vi "append_data.vi"(8 "error in (no error)":errorcluster, 10 "Current measurement #":i32, 11 "Counter in":refnum<class "Counter.lvclass">) -> (0 "error out":errorcluster, 3 "Counter out":refnum<class "Counter.lvclass">)   [LabVIEW 2013, in "Counter.lvclass"]
uses:
  Counter.lvclass
  Counter.lvclass/Counter.ctl
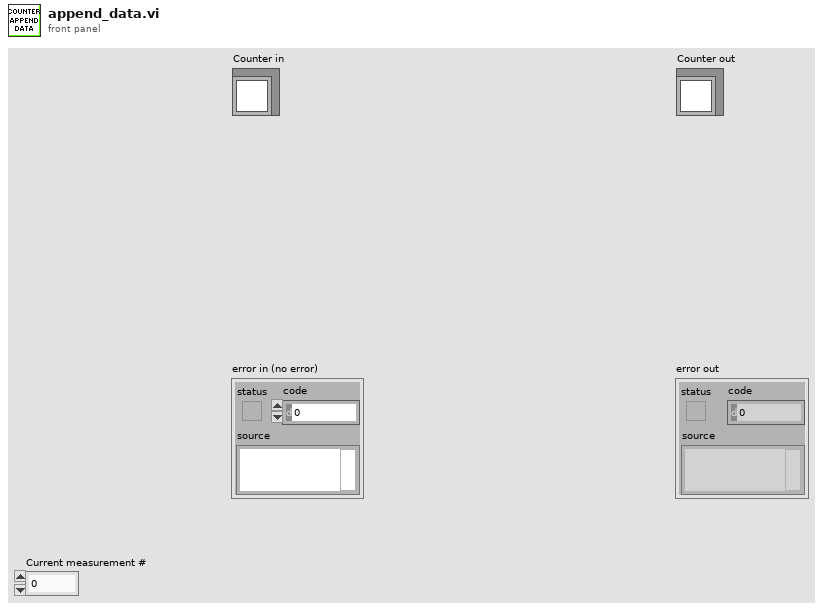
[diagram p1: front panel]
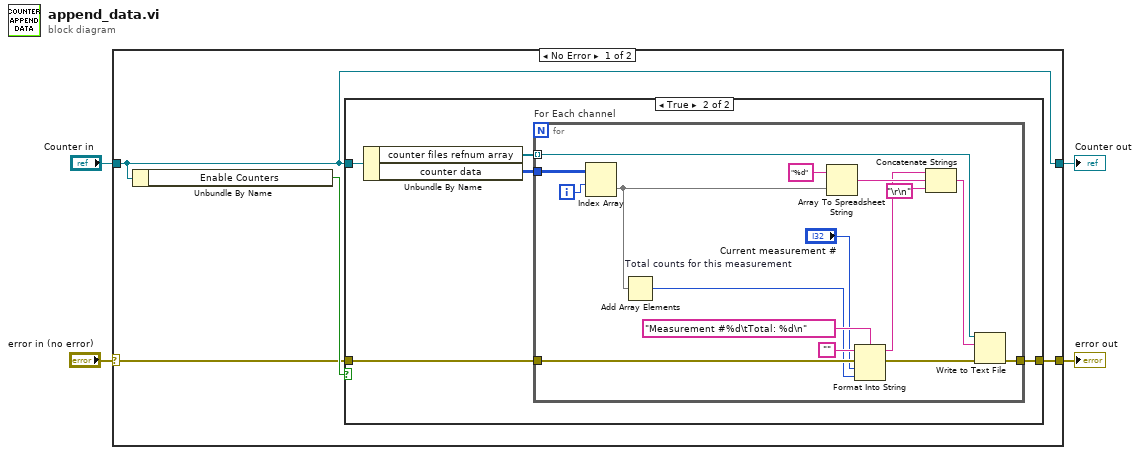
[diagram p0: block diagram]
diagram:
  n1 = case shown="No Error" "error in (no error)" {
    selector: "error in (no error)" -> [w7 w32]
    tunnel: [w5 w31] -> w2
    tunnel: "Counter in" -> [w5 w31]
    tunnel: [w6 w32] -> w1
    frame No Error {
      n2 = Unbundle By Name(w5) -> ("Enable Counters"=w8:bool)
      n3 = case shown="True" w8 {
        tunnel: w7 -> [w9 w14]
        tunnel: [w9 w13] -> w6
        tunnel: w5 -> [_ w12]
        frame False {
        }
        frame True {
          n4 = Unbundle By Name(w12) -> ("counter files refnum array"=w11:refnum<file>[], "counter data"=w10:u32[][])
          n5 = for "For Each channel" {
            tunnel: w14 -> [w30]
            tunnel: [w29] -> w13
            tunnel: w10 -> [w28]
            tunnel: w11 -> [w25] mode=indexing
            i -> [w15]
            n6 = Index Array(array=w28, index (row)=w15) -> (element=w27:u32[])  [unwired: 1 in]
            n7 = Add Array Elements "Total counts for this measurement"(numeric array=w27) -> (sum=w17:u32)
            n8 = Array To Spreadsheet String(array=w27, 3:"%d" ("format string")) -> (spreadsheet string=w20:string)  [unwired: 1 in]
            n9 = Format Into String(format string="Measurement #%d\tTotal: %d\n", initial string="", error in=w30, "Current measurement #", w17) -> (resulting string=w19:string, error out=w24:errorcluster)
            n10 = Concatenate Strings(w19, w20, "\r\n") -> (w23:string)
            n11 = Write to Text File(file (use dialog)=w25, text=w23, error in=w24) -> (error out=w29:errorcluster)  [unwired: 1 in, 2 out]
          }
        }
      }
    }
    frame Error {
    }
  }
  "error out" <- w1
  "Counter out" <- w2
